vi "BTW_Aegis_Database_Ops.vi"(8 "Error in (no error)":errorcluster, 10 "Operation":T1(ring)=enum."Select", 11 "SQL Query":string) -> (0 "Error out":errorcluster, 2 "Rec Count":i32=11, 3 "RecordSet":string[][](array[string]))   [LabVIEW 2013]
panel:
  in  "Record data":string[](array[string])
  out "Column Names":string[](array[string])
  in  "ConnectionString":string="Driver={SQL Server};Server=BTWSQLSERVER2;Database=Fusion_Prod;Uid=Aegis;Pwd=Aegis;"
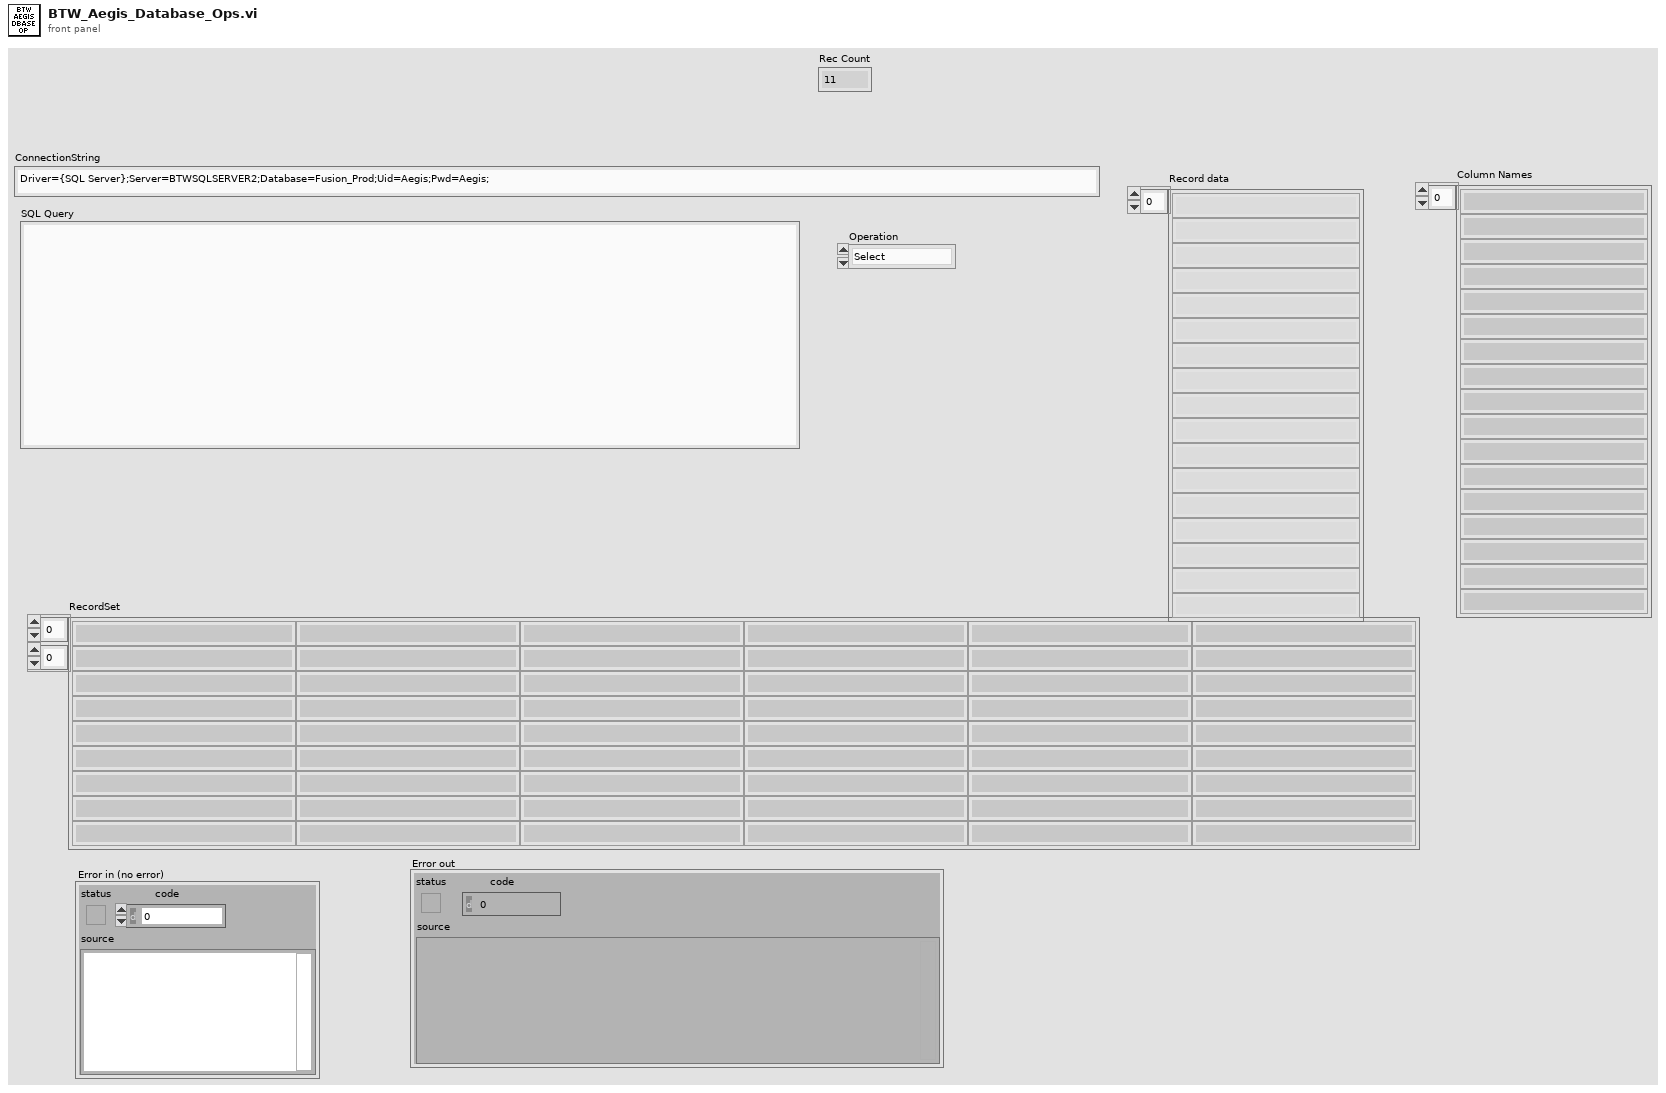
[diagram p1: front panel]
types:
  T1 = enum16{"Query", "Insert", "Select", "Dump Recs", "Get Rec Count", "Get Col Names"}
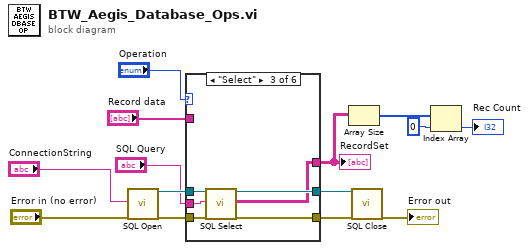
[diagram p0: block diagram]
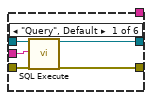
[diagram p2: hidden frame]
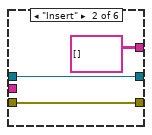
[diagram p3: hidden frame]
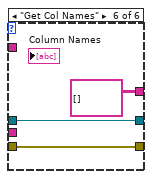
[diagram p6: hidden frame]
diagram:
  n1 = call "SQL Open.vi"("ConnectionString In"="ConnectionString", "Error in (no error)"="Error in (no error)") -> ("Connection Out"=w10:refnum<k7>, "Error out"=w9:errorcluster)  [unwired: 16 in]
  n2 = case shown="\"Select\"" "Operation" {
    tunnel: [w16 w22 w24 w29 w32 w35] -> w12
    tunnel: [w15 w21 w25 w30 w31 w33] -> w11
    tunnel: w10 -> [w18 w21 w26 w30 w31 w33]
    tunnel: w9 -> [w17 w22 w28 w29 w32 w35]
    tunnel: "SQL Query" -> [w19 _ w27 _ _ _]
    tunnel: [_ string[][] [] ("Data") w23 _ _ string[][] [] ("Data")] -> w3
    tunnel: "Record data" -> [_ _ _ _ _ _]
    frame "Query", Default {
      n3 = call "SQL Execute.vi"("Connection In"=w18, "SQL Query"=w19, "Error in (no error)"=w17) -> ("Connection Out"=w15:refnum<k7>, "Error out"=w16:errorcluster)  [unwired: 15 in]
    }
    frame "Insert" {
    }
    frame "Select" {
      n4 = call "SQL Select.vi"("Connection In"=w26, "SQL Query"=w27, "Error in (no error)"=w28) -> ("Connection Out"=w25:refnum<k7>, "Data"=w23:string[][], "Error out"=w24:errorcluster)  [unwired: 14 in]
    }
    frame "Dump Recs" {
    }
    frame "Get Rec Count" {
    }
    frame "Get Col Names" {
    }
  }
  "RecordSet" <- w3
  n5 = Array Size(array=w3) -> (size(s)=w5:i32[])
  n6 = call "SQL Close.vi"("Connection In"=w11, "Error in (no error)"=w12) -> ("Error out"=→"Error out":errorcluster)  [unwired: 17 in]
  n7 = Index Array(array=w5, index=0) -> (element=→"Rec Count":i32)
